vi "table.vi"() -> ()   [LabVIEW 2012]
panel:
  out "appended array 3":i32[](array[numeric])
  out "appended array 2":string[](array[string])
  out "Table Control":string[][](table)
  in  "Array":string[](array[string])
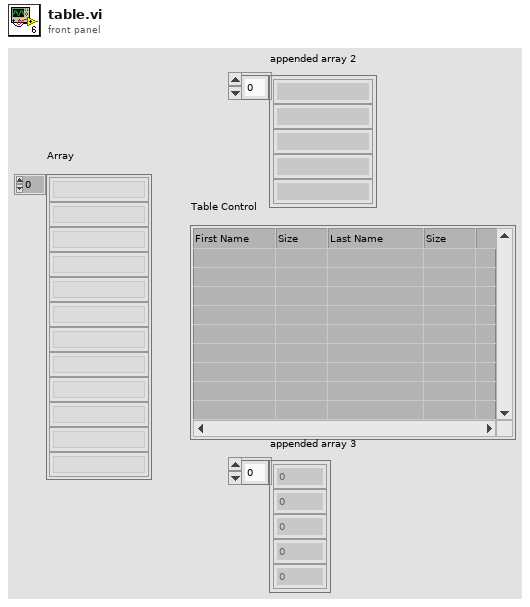
[diagram p1: front panel]
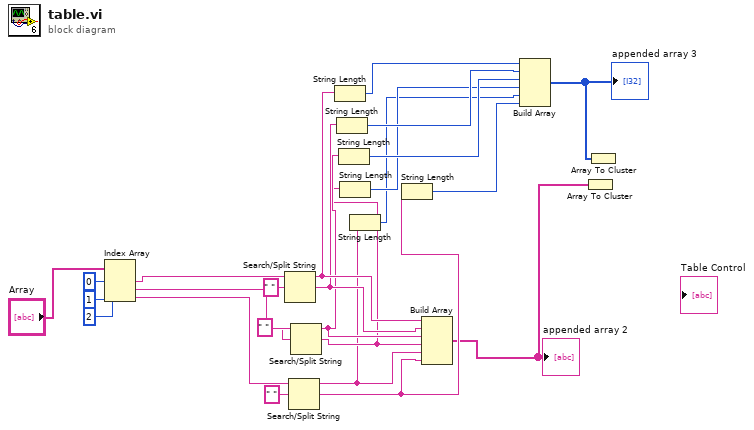
[diagram p0: block diagram]
diagram:
  n1 = Index Array(array="Array", index #1=0 ("index"), index #2=1 ("index"), index #3=2 ("index")) -> (element #1=w20:string, element #2=w19:string, element #3=w18:string)
  n2 = Search/Split String(string=w20, search string/char (-)=" ") -> (substring before match=w14:string, match + rest of string=w13:string)  [unwired: 1 in, 1 out]
  n3 = Search/Split String(string=w18, search string/char (-)=" ") -> (substring before match=w10:string, match + rest of string=w9:string)  [unwired: 1 in, 1 out]
  n4 = Search/Split String(string=w19, search string/char (-)=" ") -> (substring before match=w12:string, match + rest of string=w11:string)  [unwired: 1 in, 1 out]
  n5 = String Length(string=w14) -> (length=w8:i32)
  n6 = String Length(string=w13) -> (length=w7:i32)
  n7 = String Length(string=w12) -> (length=w6:i32)
  n8 = String Length(string=w11) -> (length=w5:i32)
  n9 = String Length(string=w10) -> (length=w4:i32)
  n10 = String Length(string=w9) -> (length=w3:i32)
  n11 = Build Array(w14, w13, w12, w11, w10, w9) -> (w1:string[])
  "appended array 2" <- w1
  n12 = Build Array(w8, w7, w6, w5, w4, w3) -> (w2:i32[])
  "appended array 3" <- w2
  n13 = Array To Cluster(array=w1) -> ()  [unwired: 1 out]
  n14 = Array To Cluster(array=w2) -> ()  [unwired: 1 out]
